vi "SC_schleife_Kelvinox.vi"   [LabVIEW 2019]
uses:
  Monitors/Utility/Monitor Communication/Kelvinox/Kelvinox_Control.ctl
  Global/Global Variables/global.vi
  Global/Global Variables/Data_Display_global.vi
  Instrument_Setup.vi
types:
  T1 = typedef "Kelvinox_Control.ctl" = cluster{"T-Setpoint-Manual":dbl, "Rate (K/min)":dbl, "Change T Control Status":bool, "Emergency Stop":bool, "Set Setpoint":bool}
  T2 = typedef "Kelvinox_Status.ctl" = cluster{"V1":bool, "V2":bool, "Dump":u16, "V4":bool, "V5":bool, "V9":bool, "P1":dbl, "P2":dbl, "P3":dbl, "P4":dbl, "P5":dbl, "Turbo":bool, "Forepump":bool, "speed":dbl, "Sorb":dbl, "1K Pot":dbl, "Still":dbl, "Cold\nPlate":dbl, "MC":dbl, "4K":dbl, "Sample":dbl, "T-Setpoint":dbl, "MC Heater":dbl, "Still Heater":dbl, "Sorb Heater":dbl, "T Control active":bool, "Sorb Res":dbl, "1K Pot Res":dbl, "Still Res":dbl, "Cold Plate Res":dbl, "MC Res":dbl, "4K Res":dbl, "Sample Res":dbl, "Ramping":bool}
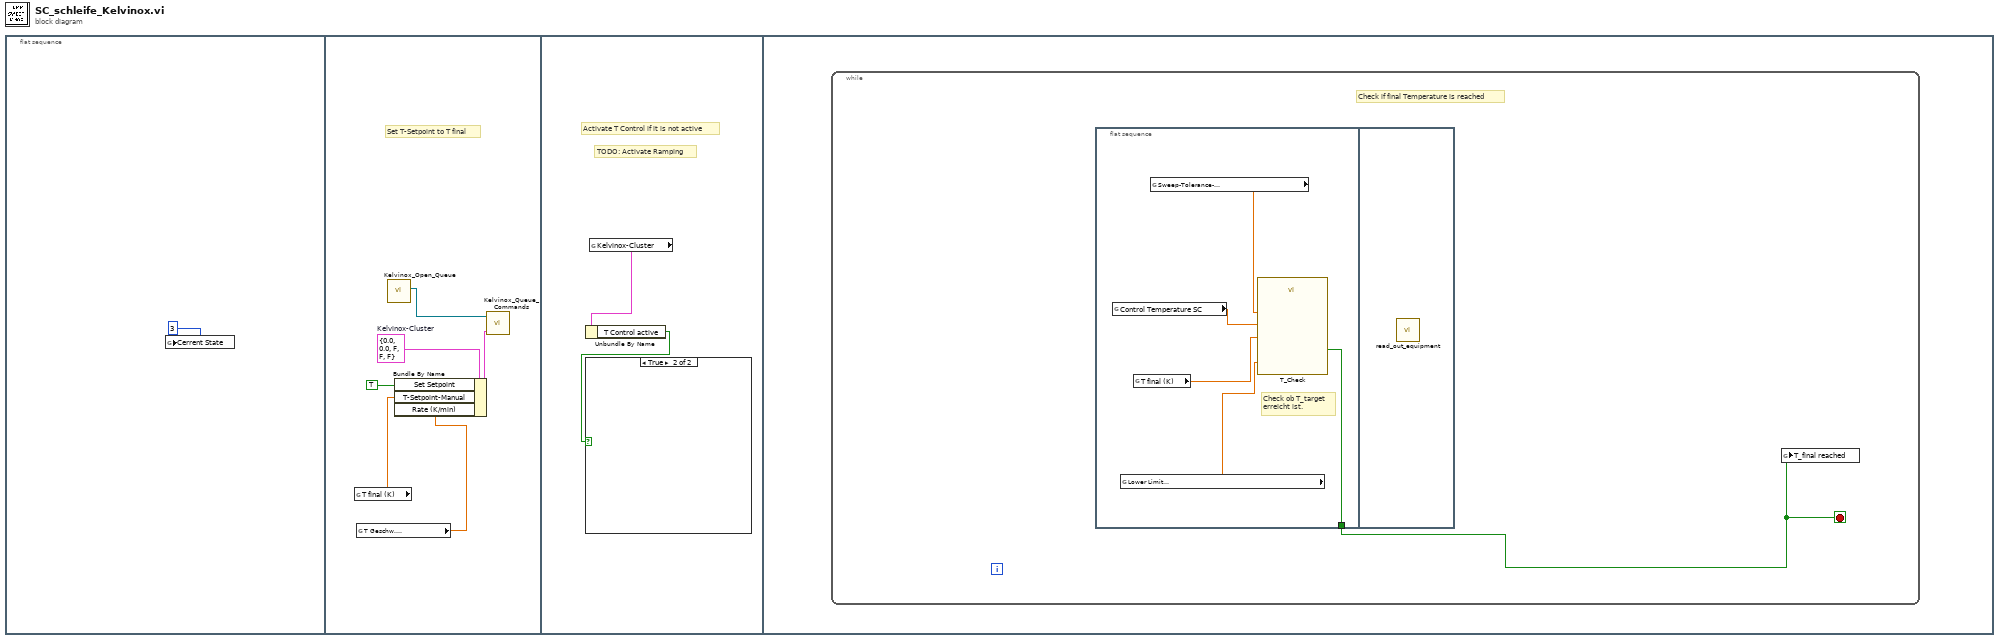
[diagram p0: block diagram]
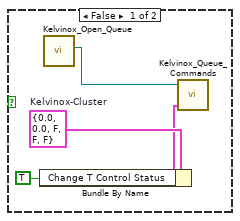
[diagram p2: hidden frame]
diagram:
  n1 = flat-sequence {
    frame #0 {
      n2 = global write "global.vi" "Cerrent State"(3) -> ()
    }
    frame #1 {
      w6 = T1 {"T-Setpoint-Manual"=0.0, "Rate (K/min)"=0.0, "Change T Control Status"=FALSE, "Emergency Stop"=FALSE, "Set Setpoint"=FALSE}  # Kelvinox-Cluster
      # "Set T-Setpoint to T final"
      n3 = global read "global.vi" "T final (K)"() -> (w3:dbl)
      n4 = global read "global.vi" "T Geschw. \n(K/min)"() -> (w2:dbl)
      n5 = call "Kelvinox_Open_Queue.vi"() -> ("queue out"=w7:refnum<queue>)  [unwired: 10 in, 1 out]
      n6 = Bundle By Name(cluster=w6, "Set Setpoint"=TRUE, "T-Setpoint-Manual"=w3, "Rate (K/min)"=w2) -> (w5:T1)
      n7 = call "Kelvinox_Queue_Commands.vi"("Control"=w5, "Queue"=w7) -> ()  [unwired: 1 in, 1 out]
    }
    frame #2 {
      # "TODO: Activate Ramping"
      # "Activate T Control if it is not active"
      n8 = global read "Data_Display_global.vi" "Kelvinox-Cluster"() -> (w9:T2)
      n9 = Unbundle By Name(w9) -> ("T Control active"=w8:bool)
      n10 = case shown="True" w8 {
        frame False {
          w12 = T1 {"T-Setpoint-Manual"=0.0, "Rate (K/min)"=0.0, "Change T Control Status"=FALSE, "Emergency Stop"=FALSE, "Set Setpoint"=FALSE}  # Kelvinox-Cluster
          n11 = Bundle By Name(cluster=w12, "Change T Control Status"=TRUE) -> (w11:T1)
          n12 = call "Kelvinox_Open_Queue.vi"() -> ("queue out"=w13:refnum<queue>)  [unwired: 10 in, 1 out]
          n13 = call "Kelvinox_Queue_Commands.vi"("Control"=w11, "Queue"=w13) -> ()  [unwired: 1 in, 1 out]
        }
        frame True {
        }
      }
    }
    frame #3 {
      n14 = while {
        stop <- w14 stop-if-true
        # "Check if final Temperature is reached"
        n15 = flat-sequence {
          tunnel: [w16] -> w14
          frame #0 {
            # "Check ob T_target\nerreicht ist."
            n16 = global read "Data_Display_global.vi" "Control Temperature SC"() -> (w19:dbl)
            n17 = global read "Instrument_Setup.vi" "Lower Limit\nSweep-Tolerance-\nTemperature (K)"() -> (w15:dbl)
            n18 = global read "global.vi" "T final (K)"() -> (w18:dbl)
            n19 = global read "Instrument_Setup.vi" "Sweep-Tolerance-\nTemperature (%)"() -> (w17:dbl)
            n20 = call "T_Check.vi"("Lower Limit Sweep\nTolerance (K)"=w15, "T_target (K)"=w18, "Sweep\nTolerance %"=w17, "T_in"=w19) -> ("= T target"=w16:bool)
          }
          frame #1 {
            n21 = call "read_out_equipment.vi"() -> ()  [unwired: 1 in]
          }
        }
        n22 = global write "Data_Display_global.vi" "T_final reached"(w14) -> ()
      }
    }
  }
